vi "_Write.vi"(5 "Maximum File Size (Bytes)":i64, 6 "File Extension":string="csv", 7 "Maximum File Count":i32, 8 "Error In":errorcluster, 9 "Enable Calendar Tree":bool=TRUE, 10 "Messages":T1[](array[typedef]), 11 "Log In":refnum<file>) -> (0 "Error Out":errorcluster, 3 "Log Out":refnum<file>)   [LabVIEW 2015, in "Logger.lvlib" / "File.lvlib"]
uses:
  File.lvlib
  Public/Controls/Message.ctl
  Public/Controls/Tag.ctl
  Logger.lvlib
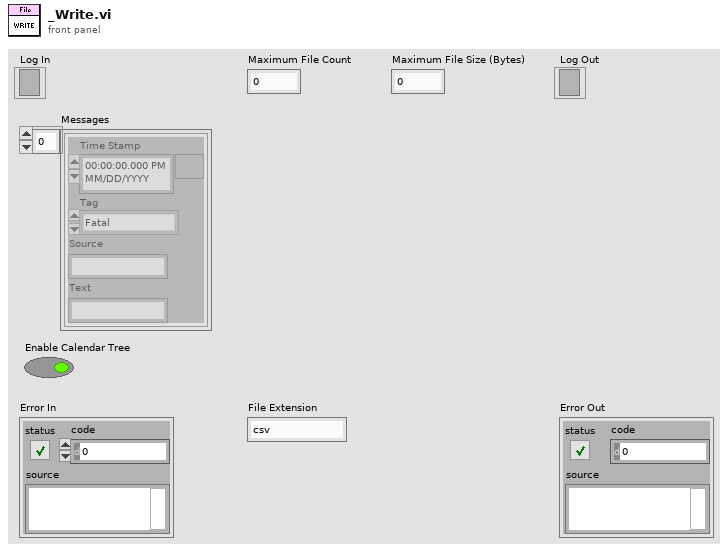
[diagram p1: front panel]
types:
  T1 = typedef "Logger.lvlib/Message.ctl" = cluster{"Time Stamp":timestamp, "Tag":T2, "Source":string, "Text":string}
  T2 = typedef "Logger.lvlib/Tag.ctl" = enum16{"Fatal", "Error", "Warn", "Info", "Debug", "Trace"}
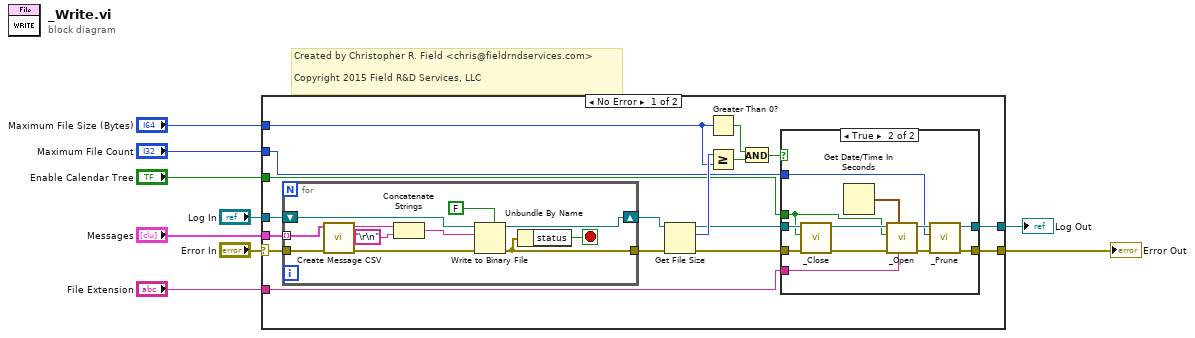
[diagram p0: block diagram]
diagram:
  # "Created by Christopher R. Field <chris@fieldrndservices.com>\n\nCopyright 2015 Field R&D Services, LLC"
  n1 = case shown="No Error" "Error In" {
    selector: "Error In" -> [w25 w52]
    tunnel: "Log In" -> [w26 w53]
    tunnel: "Messages" -> [w24 _]
    tunnel: [w14 w53] -> w6
    tunnel: [w13 w52] -> w5
    tunnel: "Maximum File Size (Bytes)" -> [w15 _]
    tunnel: "Enable Calendar Tree" -> [w12 _]
    tunnel: "Maximum File Count" -> [w11 _]
    tunnel: "File Extension" -> [w10 _]
    frame No Error {
      n2 = for {
        tunnel: w25 -> [w47]
        tunnel: w24 -> [w44] mode=indexing
        shift-right: [w42] -> w17
        shift-left: w26 -> [w49]
        tunnel: [w41] -> w16
        stop <- w43 stop-if-true
        n3 = call "Create Message CSV.vi"("Error In"=w47, "Message"=w44) -> ("Error Out"=w46:errorcluster, "CSV"=w45:string)  [unwired: 8 in]
        n4 = Concatenate Strings(w45, "\r\n") -> (w50:string)
        n5 = Write to Binary File(file (use dialog)=w49, data=w50, error in=w46, 5:FALSE ("prepend array or string size? (T)")) -> (refnum out=w42:refnum<file>, error out=w41:errorcluster)  [unwired: 2 in, 1 out]
        n6 = Unbundle By Name(w41) -> ("status"=w43:bool)
      }
      n7 = Get File Size(file=w17, error in=w16) -> (refnum out=w19:refnum<file>, size (in bytes)=w21:i64, 0:w18:errorcluster)
      n8 = Greater Than 0?(x=w15) -> (x > 0?=w22:bool)
      n9 = Greater Or Equal?(x=w21, y=w15) -> (x >= y?=w23:bool)
      n10 = And(x=w22, y=w23) -> (x .and. y?=w20:bool)
      n11 = case shown="True" w20 {
        tunnel: [w28 w32] -> w14
        tunnel: [w27 w33] -> w13
        tunnel: w19 -> [w28 w39]
        tunnel: w18 -> [w27 w38]
        tunnel: w12 -> [_ w30]
        tunnel: w11 -> [_ w31]
        tunnel: w10 -> [_ w29]
        frame False {
        }
        frame True {
          n12 = call "_Close.vi"("Error In"=w38, "Enable Calendar Tree"=w30, "Log In"=w39) -> ("Error Out"=w37:errorcluster, "Base Log Folder"=w36:path)  [unwired: 7 in]
          n13 = Get Date/Time In Seconds() -> (seconds since 1Jan1904=w40:timestamp)
          n14 = call "_Open.vi"("File Extension"=w29, "Start Time Stamp"=w40, "Error In"=w37, "Enable Calendar Tree"=w30, "Base Folder"=w36) -> ("Error Out"=w34:errorcluster, "Log Out"=w35:refnum<file>)  [unwired: 5 in]
          n15 = call "_Prune.vi"("Error In"=w34, "Maximum File Count"=w31, "File In"=w35) -> ("Error Out"=w33:errorcluster, "File Out"=w32:refnum<file>)  [unwired: 7 in]
        }
      }
    }
    frame Error {
    }
  }
  "Log Out" <- w6
  "Error Out" <- w5
